vi "TestRunner.vi"() -> ()   [LabVIEW 2014]
uses:
  Private/Class/meth.Constructor.vi
  Private/Class/meth.SetStreamReader.vi
  Private/Class/meth.ExecFunction.vi
  Private/Class/meth.Destructor.vi
  GLue.lvlib
panel:
  in  "Continue":bool
  out "Output":string
  out "error out":errorcluster
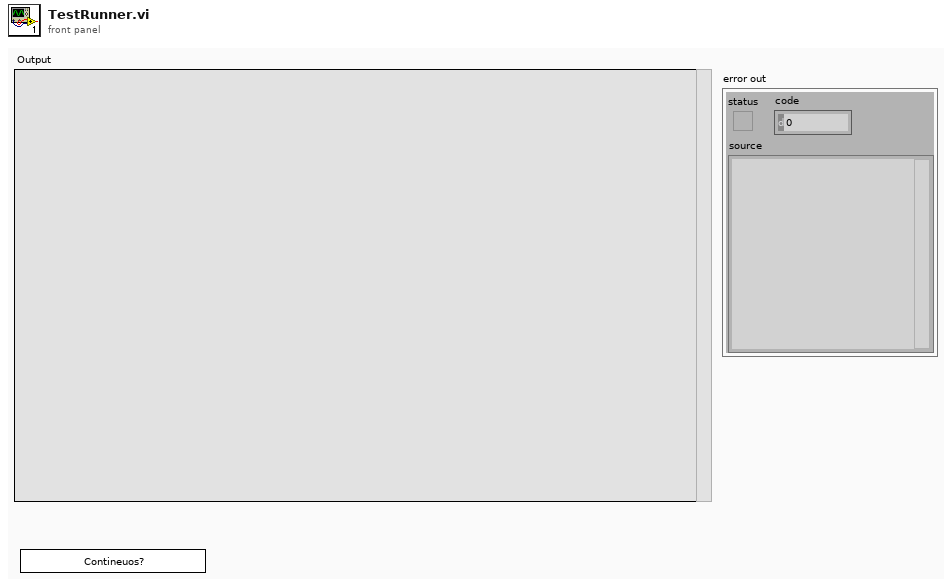
[diagram p1: front panel]
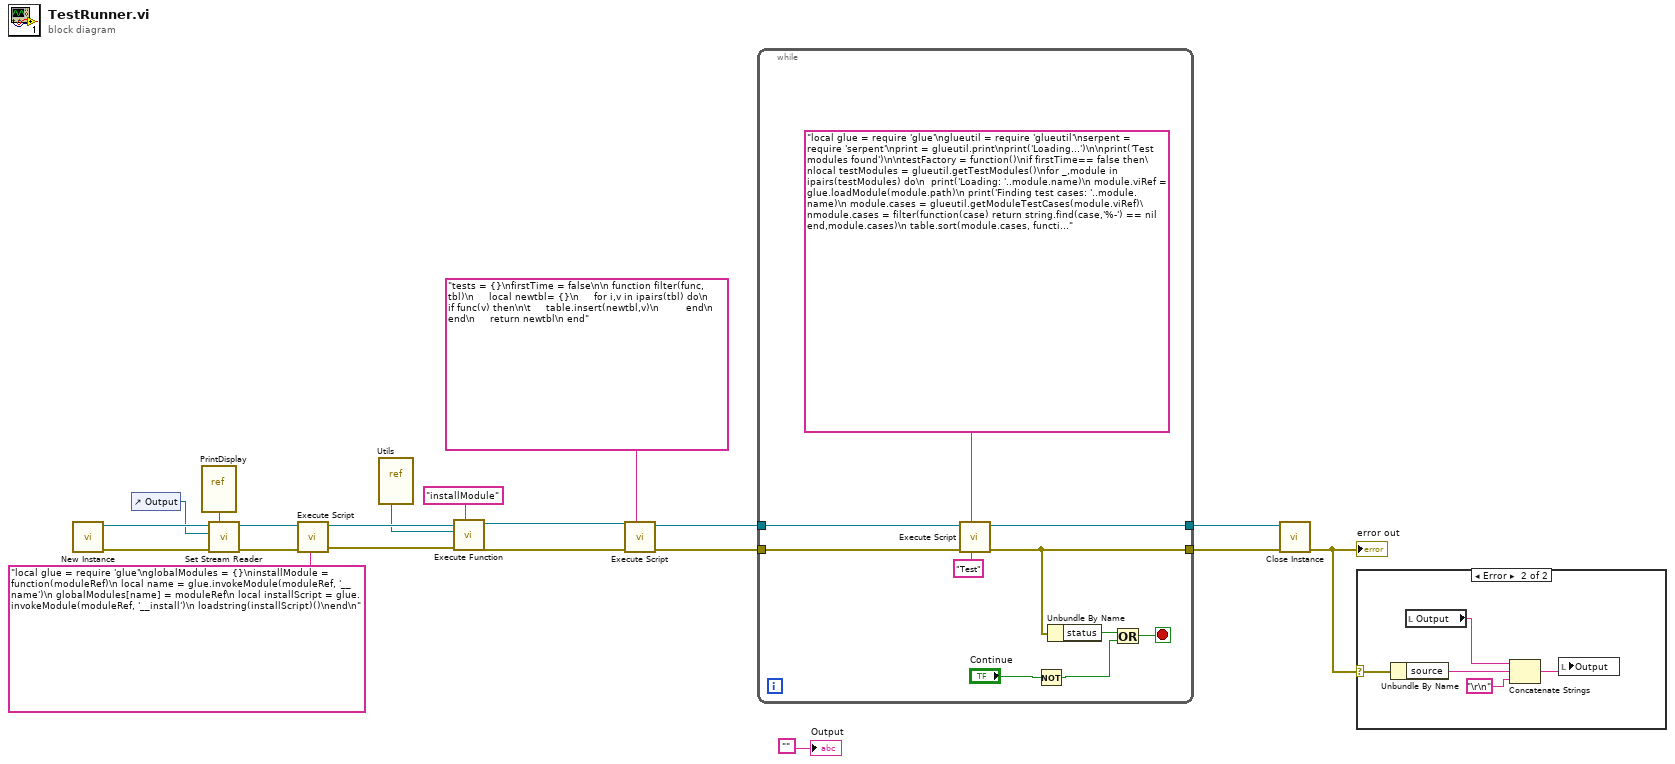
[diagram p0: block diagram]
diagram:
  n1 = call "New Instance.vi"() -> ("error out"=w13:errorcluster, "GLue out"=w12:refnum<class "class.GLue.lvclass">)  [unwired: 10 in]
  n2 = control-ref of="Output"() -> (w10:refnum<vi>)
  n3 = vi-ref "PrintDisplay.vi"() -> (w11:refnum<vi>)
  n4 = call "Set Stream Reader.vi"("StreamReader"=w11, "error in"=w13, "UserData"=w10, "GLue in"=w12) -> ("error out"=w9:errorcluster, "GLue out"=w8:refnum<class "class.GLue.lvclass">)  [unwired: 6 in]
  n5 = call "Execute Script.vi"("Script"="local glue = require 'glue'\nglobalModules = {}\ninstallModule = function(moduleRef)\n local name = glue.invokeModule(moduleRef, '__name')\n globalModules[name] = moduleRef\n local installScript = glue.invokeModule(moduleRef, '__install')\n loadstring(installScript)()\nend\n", "error in"=w9, "GLue in"=w8) -> ("error out"=w6:errorcluster, "GLue out"=w5:refnum<class "class.GLue.lvclass">)  [unwired: 6 in, 1 out]
  n6 = vi-ref "Utils.vi"() -> (w1:refnum<vi>)
  n7 = call "Execute Function.vi"("Function Name"="installModule", "error in"=w6, "Argument Data"=w1, "GLue in"=w5) -> ("error out"=w3:errorcluster, "GLue out"=w4:refnum<class "class.GLue.lvclass">)  [unwired: 5 in, 1 out]
  n8 = call "Execute Script.vi"("Script"="tests = {}\nfirstTime = false\n\n function filter(func, tbl)\n     local newtbl= {}\n     for i,v in ipairs(tbl) do\n         if func(v) then\n\t     table.insert(newtbl,v)\n         end\n     end\n     return newtbl\n end", "error in"=w3, "GLue in"=w4) -> ("error out"=w15:errorcluster, "GLue out"=w16:refnum<class "class.GLue.lvclass">)  [unwired: 6 in, 1 out]
  n9 = while {
    tunnel: [w30] -> w20
    tunnel: [w27] -> w19
    tunnel: w15 -> [w22]
    tunnel: w16 -> [w21]
    stop <- w23 stop-if-true
    n10 = call "Execute Script.vi"("Name"="Test", "Script"="local glue = require 'glue'\nglueutil = require 'glueutil'\nserpent = require 'serpent'\nprint = glueutil.print\nprint('Loading...')\n\nprint('Test modules found')\n\ntestFactory = function()\nif firstTime== false then\nlocal testModules = glueutil.getTestModules()\nfor _,module in ipairs(testModules) do\n  print('Loading: '..module.name)\n module.viRef = glue.loadModule(module.path)\n print('Finding test cases: '..module.name)\n module.cases = glueutil.getModuleTestCases(module.viRef)\nmodule.cases = filter(function(case) return string.find(case,'%-') == nil end,module.cases)\n table.sort(module.cases, function(a,b)\n  return string.lower(a) < string.lower(b) end)\n\n print('Adding: '..module.name)\n globalModules[module.name] = module.viRef\n table.insert(tests, module)\nend\nfirstTime = true\nreturn tests\nelse\nreturn tests\nend\nend\n\nlocal numTests = 0\n\n-- test runner --\nprint('testing...')\ntestToRun = testFactory()\nfor _,mod in ipairs(testToRun) do\n  print('>> ' .. mod.name)\n  for _,test in ipairs(mod.cases) do   \n    local res,msg = pcall(function() \n          glue.invokeModule(globalModules[mod.name],test)\n          print( 'pass -- ' .. test)\n          numTests = numTests + 1\n        end)\n    if res ~= true then\n     local failedTest = 'fail -- ' .. test\n     print(failedTest)\n     print(string.rep('^',#failedTest)..'\\n'..msg..'\\n')\n     return\n    end\n  end\n  print('')\nend\n\nprint(\"\\nNumber of tests: \" .. numTests)\n", "error in"=w22, "GLue in"=w21) -> ("error out"=w27:errorcluster, "GLue out"=w30:refnum<class "class.GLue.lvclass">)  [unwired: 5 in, 1 out]
    n11 = Not(x="Continue") -> (.not. x?=w24:bool)
    n12 = Unbundle By Name(w27) -> ("status"=w26:bool)
    n13 = Or(x=w26, y=w24) -> (x .or. y?=w23:bool)
  }
  n14 = call "Close Instance.vi"("error in"=w19, "GLue in"=w20) -> ("error out"=w18:errorcluster)  [unwired: 9 in]
  "error out" <- w18
  n15 = case shown="Error" w18 {
    selector: w18 -> [_ w35]
    frame No Error {
    }
    frame Error {
      n16 = Unbundle By Name(w35) -> ("source"=w33:string)
      n17 = local read "Output"() -> (w32:string)
      n18 = Concatenate Strings(w32, w33, "\r\n") -> (w31:string)
      n19 = local write "Output"(w31) -> ()
    }
  }
  "Output" <- ""
